vi "AvarageDetector.vi"(7 "avgIn":bool[][](array[boolean])) -> (8 "avgOut":bool[][](array[boolean]), 15 "OK":bool=TRUE)   [LabVIEW 2009]
panel:
  in  "Avg 4":bool[](array[boolean])=[FALSE, FALSE, TRUE, TRUE, FALSE, FALSE, TRUE, FALSE]
  in  "Avg 3":bool[](array[boolean])=[FALSE, FALSE, FALSE, TRUE, FALSE, FALSE, FALSE, FALSE]
  in  "Avg 2":bool[](array[boolean])=[FALSE, FALSE, FALSE, FALSE, FALSE, FALSE, FALSE, FALSE]
  in  "Avg 1":bool[](array[boolean])=[TRUE, FALSE, FALSE, TRUE, TRUE, FALSE, FALSE, FALSE]
  in  "OK Button":bool
  in  "Cancel Button":bool
  # "1"
  # "2"
  # "3"
  # "4"
  # "5"
  # "6"
  # "7"
  # "8"
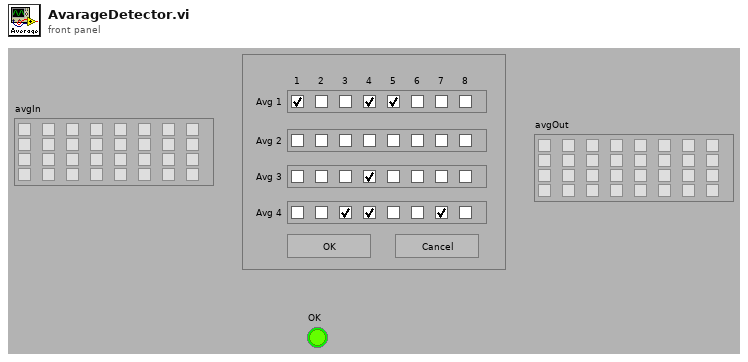
[diagram p1: front panel]
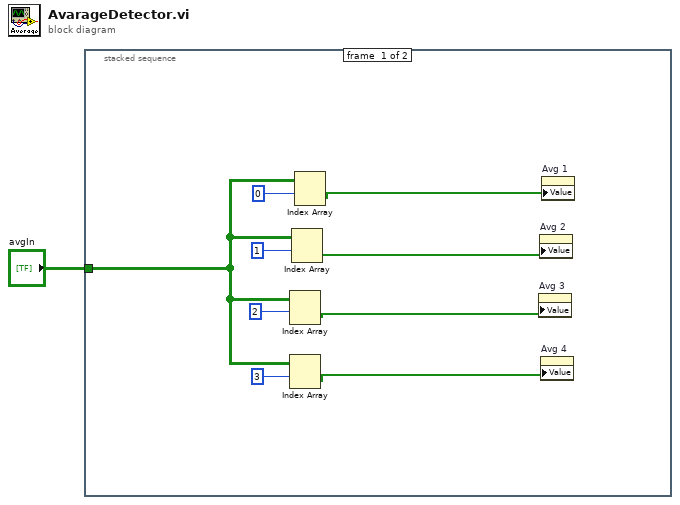
[diagram p0: block diagram]
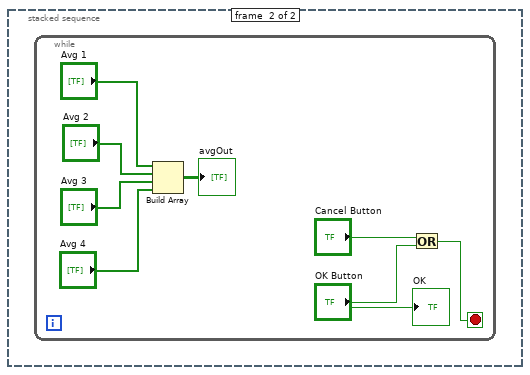
[diagram p2: hidden frame]
diagram:
  n1 = stacked-sequence {
    tunnel: "avgIn" -> [w2 _]
    frame #0 {
      n2 = Index Array(array=w2, index (row)=2) -> (element=w4:bool[])  [unwired: 1 in]
      n3 = Index Array(array=w2, index (row)=3) -> (element=w3:bool[])  [unwired: 1 in]
      n4 = Index Array(array=w2, index (row)=1) -> (element=w5:bool[])  [unwired: 1 in]
      n5 = Index Array(array=w2, index (row)=0) -> (element=w6:bool[])  [unwired: 1 in]
      n6 = property on="Avg 3" class="Arr (strict)"("Value"=w4) -> ()  [unwired: 2 in, 2 out]
      n7 = property on="Avg 2" class="Arr (strict)"("Value"=w5) -> ()  [unwired: 2 in, 2 out]
      n8 = property on="Avg 4" class="Arr (strict)"("Value"=w3) -> ()  [unwired: 2 in, 2 out]
      n9 = property on="Avg 1" class="Arr (strict)"("Value"=w6) -> ()  [unwired: 2 in, 2 out]
    }
    frame #1 {
      n10 = while {
        stop <- w16 stop-if-true
        n11 = Build Array("Avg 1", "Avg 2", "Avg 3", "Avg 4") -> (→"avgOut":bool[][])
        n12 = Or(x="Cancel Button", y="OK Button") -> (x .or. y?=w16:bool)
        "OK" <- "OK Button"
      }
    }
  }
